vi "read_file.vi"() -> ()   [LabVIEW 2015]
panel:
  out "Array":dbl[][](array[numeric])
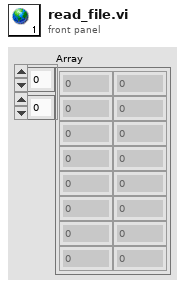
[diagram p1: front panel]
diagram:
